vi "Read current file list.vi"(8 "error in":errorcluster, 11 "VI modification collection in":refnum<class "VI modification collection.lvclass">) -> (0 "error out":errorcluster, 2 "current file list":path[](array[path]), 3 "VI modification collection out":refnum<class "VI modification collection.lvclass">)   [LabVIEW 2013, in "VI modification collection.lvclass"]
uses:
  VI modification collection.lvclass
  VI modification collection.lvclass/VI modification collection.ctl
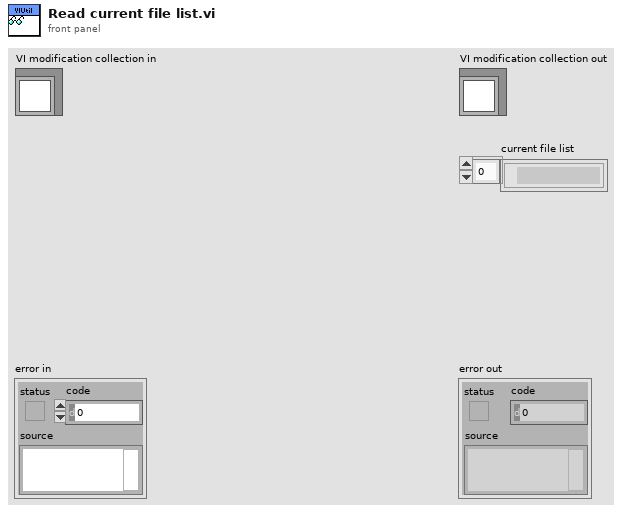
[diagram p1: front panel]
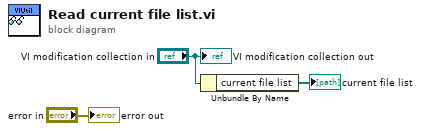
[diagram p0: block diagram]
diagram:
  n1 = Unbundle By Name("VI modification collection in") -> ("current file list"=→"current file list":path[])
  "error out" <- "error in"
  "VI modification collection out" <- "VI modification collection in"
